vi "Facade.vi"(0 "Data In":T6, 2 "Display State In":T4, 3 "Container State":T5) -> (6 "Data Out":T6, 7 "Display State Out":T4, 8 "Action":T3)   [LabVIEW 2020, in "Channel.xctl"]
uses:
  Channel.xctl
  Data.vi
  Classes/Channel/Channel.lvclass
  <vilib>/_xctls/Container State.ctl
  State.vi
  <vilib>/_xctls/Action.ctl
  Waveforms/Waveform/Waveform.xctl
  Classes/Waveforms/Waveform/Waveform.lvclass
  D:/Development/epl-vi-lib/Koop/KObject Class/KObject.lvclass
  Level/Level.xctl
  Classes/Level/Level.lvclass
  Gate/Gate.xctl
  Classes/Gate/Gate.lvclass
  Filter/Filter.xctl
  Classes/Filter/Filter.lvclass
  Modulations/AM/AM.xctl
  Classes/Modulations/AM/AM.lvclass
  Utility VIs/Buttons/KCheckmarkBoolean 2.ctl
  Classes/Channel/Channel.lvclass/Channel.ctl
  Classes/Channel/Write Destination.vi
  Classes/Channel/Write Level.vi
  Classes/Channel/Write Filter.vi
  Classes/Channel/Write Gate.vi
  Classes/Channel/Write AM.vi
  Classes/Channel/Write Invert.vi
  Classes/Channel/Write AltPol.vi
  Classes/Channel/Write Persist.vi
  Classes/Channel/Read Waveform.vi
  Classes/Channel/Read Level.vi
  Classes/Channel/Read Gate.vi
  Classes/Channel/Read Filter.vi
  Classes/Channel/Read AM.vi
  Classes/Channel/Read Invert.vi
  Classes/Channel/Read AltPol.vi
  Classes/Channel/Read Persist.vi
  Classes/Channel/Read Destination.vi
  <vilib>/_xctls/XControlSupport.lvlib
  Koop/KObject Class/KObject.lvclass
panel:
  in  "Destination":u16(ring) caption="is"
  in  "Tabs":T1(tab)
  in  "Waveform":refnum<class "Waveform.lvclass">(xcontrol)
  in  "Filter":refnum<class "Filter.lvclass">(xcontrol)
  in  "Level":refnum<class "Level.lvclass">(xcontrol)
  in  "Gate":refnum<class "Gate.lvclass">(xcontrol)
  in  "AM":refnum<class "AM.lvclass">(xcontrol)
  in  "Fade out (ms)":dbl min=0.0
  in  "Fade in (ms)":dbl min=0.0
  in  "Persist":T2
  in  "Invert":T2
  in  "Alternate polarity":T2
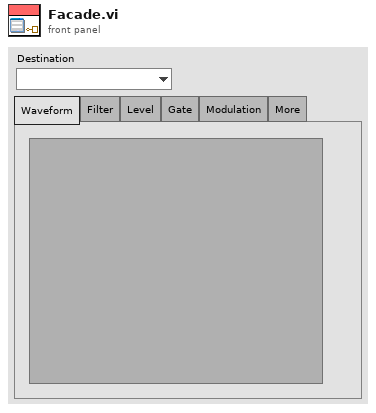
[diagram p1: front panel]
types:
  T1 = enum32{"Waveform", "Filter", "Level", "Gate", "Modulation", "More"}
  T2 = typedef "KCheckmarkBoolean 2.ctl" = bool
  T3 = typedef "XControlSupport.lvlib/Action.ctl" = cluster{"Data Changed?":bool, "State Changed?":bool, "Action Name":string}
  T4 = typedef "Channel.xctl/State.vi" = cluster{"action":string, "Destinations":string[]}
  T5 = typedef "XControlSupport.lvlib/Container State.ctl" = cluster{"Indicator?":bool, "Run Mode?":bool, " Refnum":refnum<vi>}
  T6 = typedef "Channel.xctl/Data.vi" = refnum<class "Channel.lvclass">
  T7 = typedef "Waveform.lvclass/Attributes.ctl" = cluster{"Spectrum":bool, "Gate":bool, "Mod":bool, "Filter":bool}
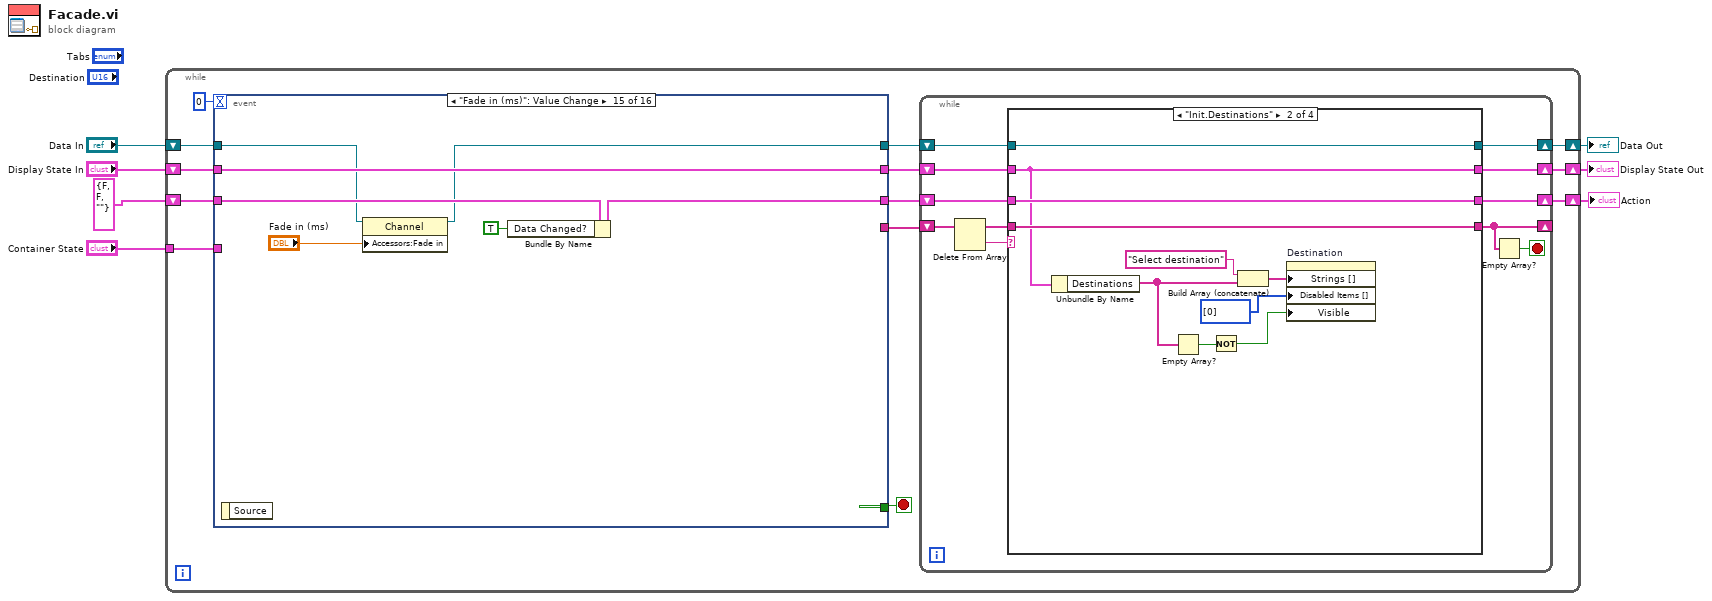
[diagram p0: block diagram]
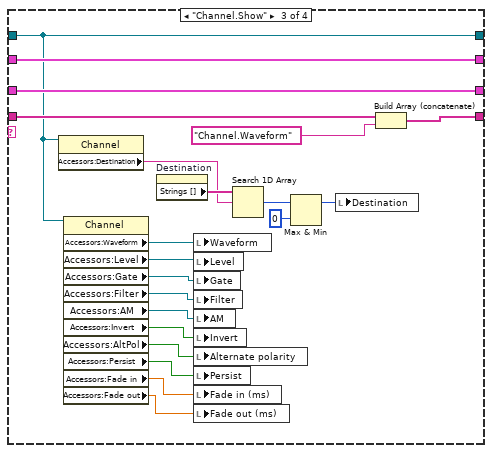
[diagram p3: hidden frame]
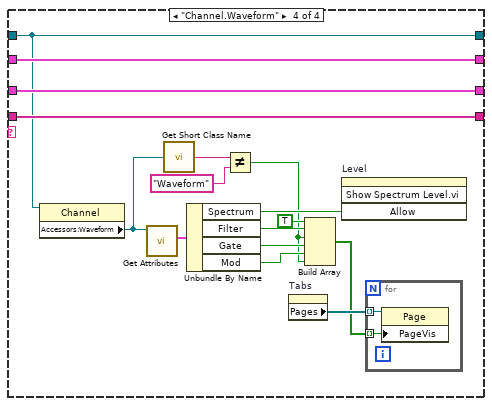
[diagram p4: hidden frame]
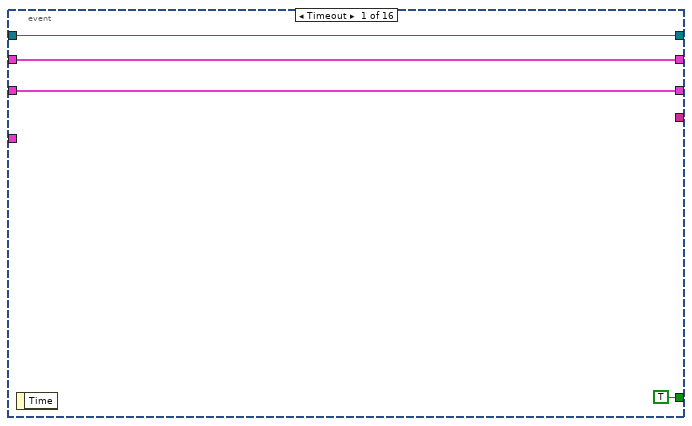
[diagram p5: hidden frame]
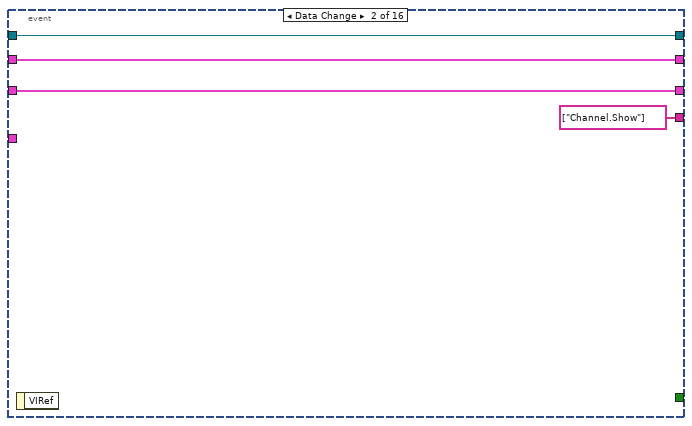
[diagram p6: hidden frame]
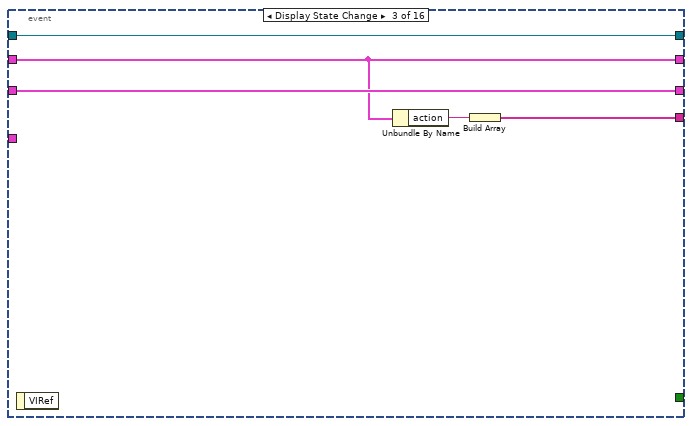
[diagram p7: hidden frame]
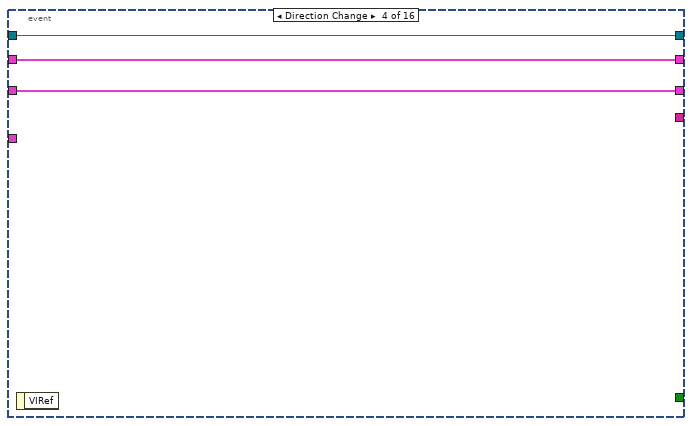
[diagram p8: hidden frame]
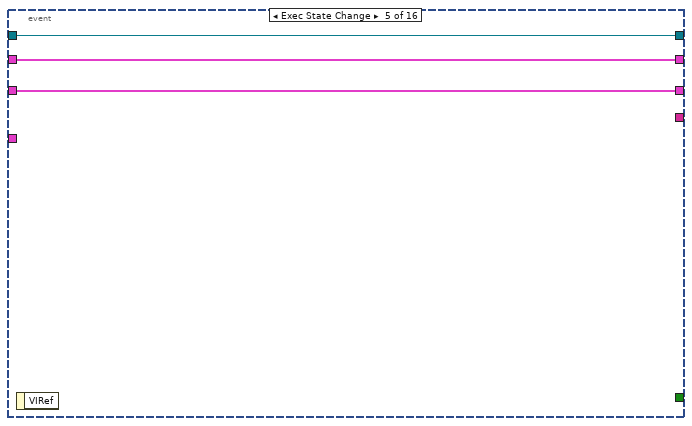
[diagram p9: hidden frame]
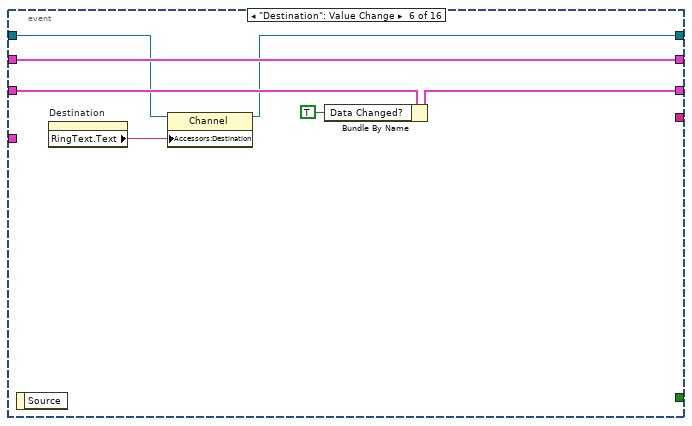
[diagram p10: hidden frame]
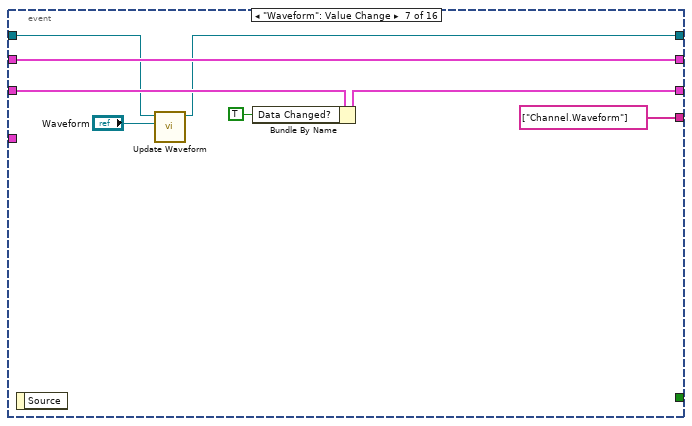
[diagram p11: hidden frame]
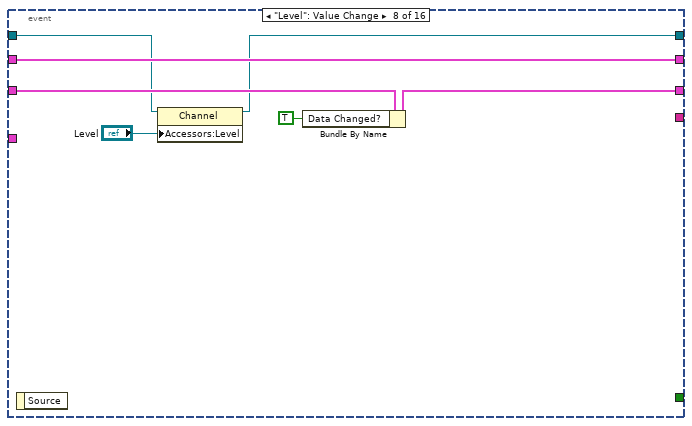
[diagram p12: hidden frame]
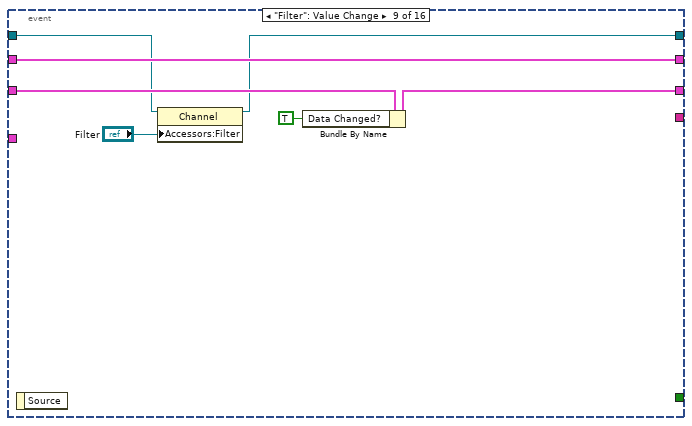
[diagram p13: hidden frame]
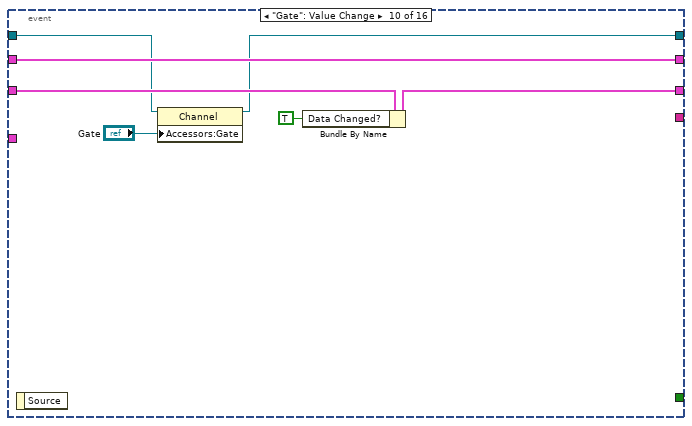
[diagram p14: hidden frame]
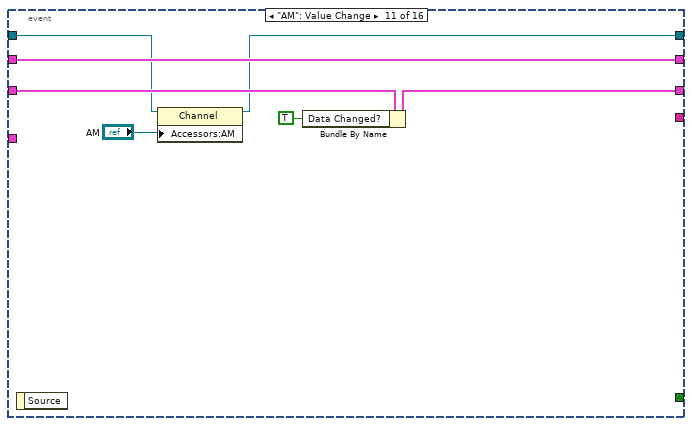
[diagram p15: hidden frame]
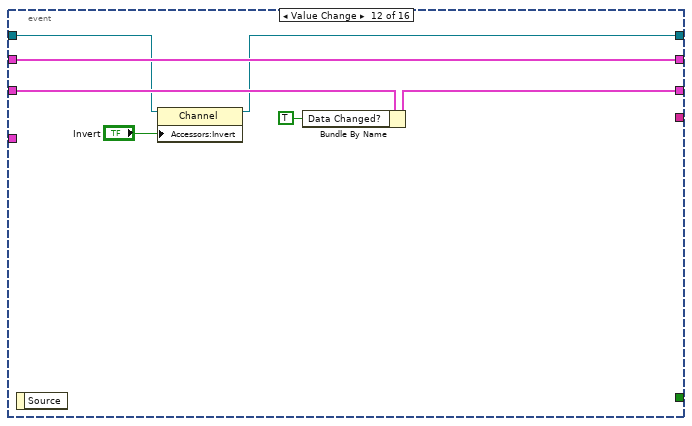
[diagram p16: hidden frame]
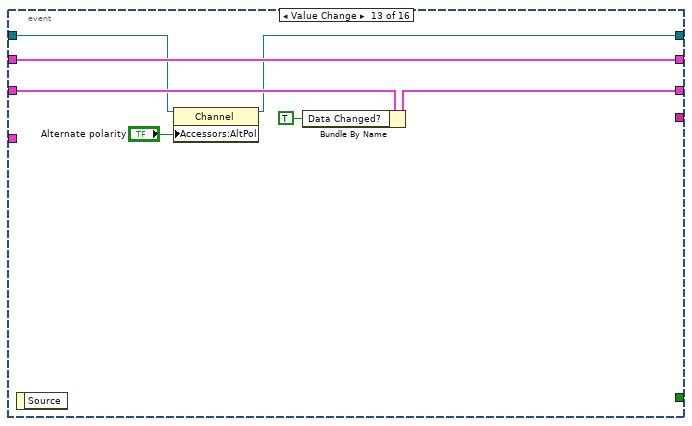
[diagram p17: hidden frame]
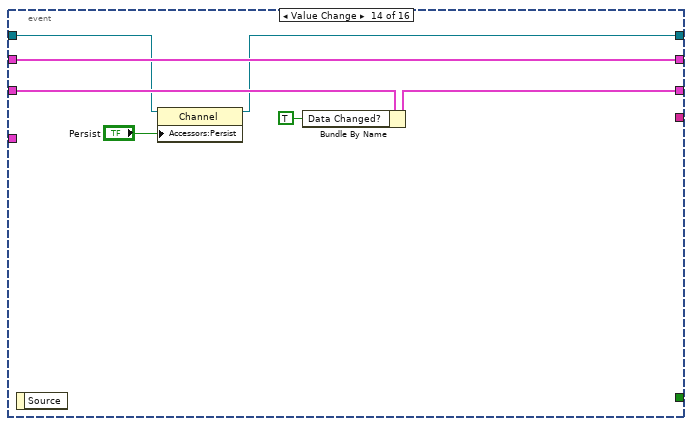
[diagram p18: hidden frame]
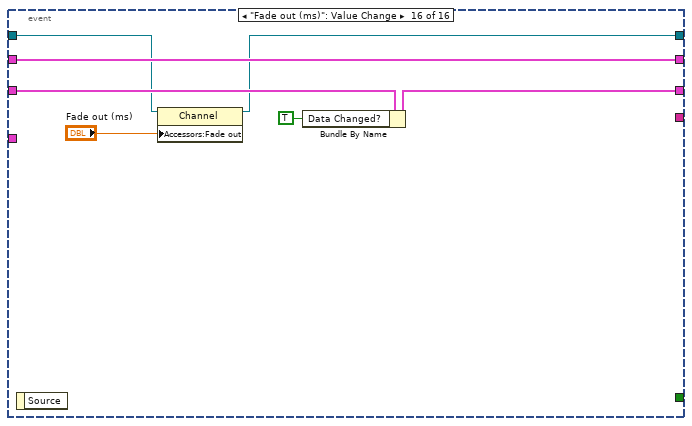
[diagram p19: hidden frame]
diagram:
  n1 = while {
    shift-right: [w9] -> w4
    shift-left: "Display State In" -> [w20]
    tunnel: "Container State" -> [w17]
    shift-right: [w10] -> w7
    shift-left: "Data In" -> [w16]
    shift-right: [w8] -> w2
    shift-left: T3 {"Data Changed?"=FALSE, "State Changed?"=FALSE, "Action Name"=""} ("Action") -> [w15]
    stop <- w19 stop-if-true
    n2 = event shown="[14] \"Fade in (ms)\": Value Change" {
      selector: _ -> [_ _ _ _ _ _ _ _ _ _ _ _ _ _ _ _]
      dyn-events: _ -> [_ _ _ _ _ _ _ _ _ _ _ _ _ _ _ _]
      timeout: 0 -> [_ _ _ _ _ _ _ _ _ _ _ _ _ _ _ _]
      tunnel: w20 -> [w86 w91 w95 w100 w103 w110 w118 w125 w132 w139 w146 w153 w160 w167 w174 w181]
      tunnel: [w86 w91 w95 w100 w103 w110 w118 w125 w132 w139 w146 w153 w160 w167 w174 w181] -> w12
      tunnel: [TRUE _ _ _ _ _ _ _ _ _ _ _ _ _ _ _] -> w19
      tunnel: w17 -> [_ _ _ _ _ _ _ _ _ _ _ _ _ _ _ _]
      tunnel: w16 -> [w85 w92 w97 w99 w102 w108 w114 w123 w130 w137 w144 w151 w158 w165 w172 w179]
      tunnel: [w85 w92 w97 w99 w102 w107 w113 w122 w129 w136 w143 w150 w157 w164 w171 w178] -> w13
      tunnel: [w87 w90 w96 w98 w101 w105 w116 w120 w128 w135 w142 w149 w156 w163 w170 w177] -> w11
      tunnel: w15 -> [w87 w90 w96 w98 w101 w109 w117 w124 w131 w138 w145 w152 w159 w166 w173 w180]
      tunnel: [_ string[] ["Channel.Show"] w93 _ _ _ string[] ["Channel.Waveform"] _ _ _ _ _ _ _ _ _] -> w14
      event Timeout {
        n3 = event-data() -> ()  [unwired: 1 in, 1 out]
      }
      event Data Change {
        n4 = event-data() -> ()  [unwired: 1 in, 1 out]
      }
      event Display State Change {
        n5 = event-data() -> ()  [unwired: 1 in, 1 out]
        n6 = Unbundle By Name(w95) -> ("action"=w94:string)
        n7 = Build Array(w94) -> (w93:string[])
      }
      event Direction Change {
        n8 = event-data() -> ()  [unwired: 1 in, 1 out]
      }
      event Exec State Change {
        n9 = event-data() -> ()  [unwired: 1 in, 1 out]
      }
      event "Destination": Value Change {
        n10 = event-data() -> ()  [unwired: 1 in, 1 out]
        n11 = property on="Destination" class="Ring (strict)"() -> ("RingText.Text"=w106:string)  [unwired: 2 in, 2 out]
        n12 = property class="Channel"(reference=w108, "Accessors:Destination"=w106) -> (reference out=w107:T6)  [unwired: 1 in, 1 out]
        n13 = Bundle By Name(cluster=w109, "Data Changed?"=TRUE) -> (w105:T3)
      }
      event "Waveform": Value Change {
        n14 = event-data() -> ()  [unwired: 1 in, 1 out]
        n15 = call "Update Waveform.vi"("Waveform"="Waveform", "Channel in"=w114) -> ("Channel out"=w113:T6)  [unwired: 8 in, 1 out]
        n16 = Bundle By Name(cluster=w117, "Data Changed?"=TRUE) -> (w116:T3)
      }
      event "Level": Value Change {
        n17 = event-data() -> ()  [unwired: 1 in, 1 out]
        n18 = property class="Channel"(reference=w123, "Accessors:Level"="Level") -> (reference out=w122:T6)  [unwired: 1 in, 1 out]
        n19 = Bundle By Name(cluster=w124, "Data Changed?"=TRUE) -> (w120:T3)
      }
      event "Filter": Value Change {
        n20 = event-data() -> ()  [unwired: 1 in, 1 out]
        n21 = property class="Channel"(reference=w130, "Accessors:Filter"="Filter") -> (reference out=w129:T6)  [unwired: 1 in, 1 out]
        n22 = Bundle By Name(cluster=w131, "Data Changed?"=TRUE) -> (w128:T3)
      }
      event "Gate": Value Change {
        n23 = event-data() -> ()  [unwired: 1 in, 1 out]
        n24 = property class="Channel"(reference=w137, "Accessors:Gate"="Gate") -> (reference out=w136:T6)  [unwired: 1 in, 1 out]
        n25 = Bundle By Name(cluster=w138, "Data Changed?"=TRUE) -> (w135:T3)
      }
      event "AM": Value Change {
        n26 = event-data() -> ()  [unwired: 1 in, 1 out]
        n27 = property class="Channel"(reference=w144, "Accessors:AM"="AM") -> (reference out=w143:T6)  [unwired: 1 in, 1 out]
        n28 = Bundle By Name(cluster=w145, "Data Changed?"=TRUE) -> (w142:T3)
      }
      event Value Change {
        n29 = event-data() -> ()  [unwired: 1 in, 1 out]
        n30 = property class="Channel"(reference=w151, "Accessors:Invert"="Invert") -> (reference out=w150:T6)  [unwired: 1 in, 1 out]
        n31 = Bundle By Name(cluster=w152, "Data Changed?"=TRUE) -> (w149:T3)
      }
      event Value Change {
        n32 = event-data() -> ()  [unwired: 1 in, 1 out]
        n33 = property class="Channel"(reference=w158, "Accessors:AltPol"="Alternate polarity") -> (reference out=w157:T6)  [unwired: 1 in, 1 out]
        n34 = Bundle By Name(cluster=w159, "Data Changed?"=TRUE) -> (w156:T3)
      }
      event Value Change {
        n35 = event-data() -> ()  [unwired: 1 in, 1 out]
        n36 = property class="Channel"(reference=w165, "Accessors:Persist"="Persist") -> (reference out=w164:T6)  [unwired: 1 in, 1 out]
        n37 = Bundle By Name(cluster=w166, "Data Changed?"=TRUE) -> (w163:T3)
      }
      event "Fade in (ms)": Value Change {
        n38 = event-data() -> ()  [unwired: 1 in, 1 out]
        n39 = property class="Channel"(reference=w172, "Accessors:Fade in"="Fade in (ms)") -> (reference out=w171:T6)  [unwired: 1 in, 1 out]
        n40 = Bundle By Name(cluster=w173, "Data Changed?"=TRUE) -> (w170:T3)
      }
      event "Fade out (ms)": Value Change {
        n41 = event-data() -> ()  [unwired: 1 in, 1 out]
        n42 = property class="Channel"(reference=w179, "Accessors:Fade out"="Fade out (ms)") -> (reference out=w178:T6)  [unwired: 1 in, 1 out]
        n43 = Bundle By Name(cluster=w180, "Data Changed?"=TRUE) -> (w177:T3)
      }
    }
    n44 = while {
      shift-right: [w28] -> _
      shift-left: w14 -> [w31]
      shift-right: [w26] -> w10
      shift-left: w13 -> [w25]
      shift-right: [w24] -> w9
      shift-left: w12 -> [w23]
      shift-right: [w22] -> w8
      shift-left: w11 -> [w21]
      stop <- w27 stop-if-true
      n45 = Delete From Array(array=w31) -> (deleted portion=w29:string, array with subset deleted=w30:string[])  [unwired: 2 in]
      n46 = case shown="\"Init.Destinations\"" w29 {
        tunnel: w30 -> [w35 w45 w66 w82]
        tunnel: [w35 w45 w56 w82] -> w28
        tunnel: [w34 w44 w58 w79] -> w26
        tunnel: w25 -> [w34 w44 w58 w79]
        tunnel: [w33 w42 w65 w81] -> w24
        tunnel: w23 -> [w33 w42 w65 w81]
        tunnel: [w32 w43 w64 w80] -> w22
        tunnel: w21 -> [w32 w43 w64 w80]
        frame "", Default {
        }
        frame "Init.Destinations" {
          n47 = Unbundle By Name(w42) -> ("Destinations"=w38:string[])
          n48 = Empty Array?(array=w38) -> (empty?=w37:bool)
          n49 = Not(x=w37) -> (.not. x?=w36:bool)
          n50 = Build Array (concatenate)("Select destination", w38) -> (w41:string[])
          n51 = property on="Destination" class="Ring (strict)"("Strings []"=w41, "Disabled Items []"=i32[] [0], "Visible"=w36) -> ()  [unwired: 2 in, 2 out]
        }
        frame "Channel.Show" {
          n52 = property class="Channel"(reference=w58) -> ("Accessors:Destination"=w62:string)  [unwired: 1 in, 2 out]
          n53 = property class="Channel"(reference=w58) -> ("Accessors:Waveform"=w57:refnum<class "Waveform.lvclass">, "Accessors:Level"=w54:refnum<class "Level.lvclass">, "Accessors:Gate"=w53:refnum<class "Gate.lvclass">, "Accessors:Filter"=w52:refnum<class "Filter.lvclass">, "Accessors:AM"=w51:refnum<class "AM.lvclass">, "Accessors:Invert"=w50:bool, "Accessors:AltPol"=w49:bool, "Accessors:Persist"=w48:bool, "Accessors:Fade in"=w47:dbl, "Accessors:Fade out"=w46:dbl)  [unwired: 1 in, 2 out]
          n54 = property on="Destination" class="Ring (strict)"() -> ("Strings []"=w63:string[])  [unwired: 2 in, 2 out]
          n55 = local write "Waveform"(w57) -> ()
          n56 = local write "Level"(w54) -> ()
          n57 = local write "Gate"(w53) -> ()
          n58 = local write "Filter"(w52) -> ()
          n59 = local write "AM"(w51) -> ()
          n60 = local write "Invert"(w50) -> ()
          n61 = local write "Alternate polarity"(w49) -> ()
          n62 = local write "Persist"(w48) -> ()
          n63 = local write "Fade in (ms)"(w47) -> ()
          n64 = local write "Fade out (ms)"(w46) -> ()
          n65 = Search 1D Array(1D array=w63, element=w62) -> (index of element=w61:i32)  [unwired: 1 in]
          n66 = Max & Min(x=w61, y=0) -> (max(x,y)=w59:i32)  [unwired: 1 out]
          n67 = local write "Destination"(w59) -> ()
          n68 = Build Array (concatenate)(w66, "Channel.Waveform") -> (w56:string[])
        }
        frame "Channel.Waveform" {
          n69 = property class="Channel"(reference=w79) -> ("Accessors:Waveform"=w70:refnum<class "Waveform.lvclass">)  [unwired: 1 in, 2 out]
          n70 = call-dynamic "Get Attributes.vi"("Waveform in"=w70) -> ("Attributes"=w78:T7)  [unwired: 8 in, 2 out]
          n71 = call "Get Short Class Name.vi"("KObject in"=w70) -> ("Class"=w69:string)  [unwired: 4 in]
          n72 = Unbundle By Name(w78) -> ("Spectrum"=w77:bool, "Filter"=w76:bool, "Gate"=w75:bool, "Mod"=w74:bool)
          n73 = Not Equal?(x=w69, y="Waveform") -> (x != y?=w67:bool)
          n74 = property on="Tabs" class="TabCtl (strict)"() -> ("Pages"=w72:refnum<vi>[])  [unwired: 2 in, 2 out]
          n75 = Build Array(TRUE, w76, w67, w75, w74, w67) -> (w71:bool[])
          n76 = invoke on="Level" class="Level (strict)" method="Show Spectrum Level.vi"("Allow"=w77) -> ()  [unwired: 3 in, 4 out]
          n77 = for {
            tunnel: w72 -> [w84] mode=indexing
            tunnel: w71 -> [w83] mode=indexing
            n78 = property class="Page"(reference=w84, "PageVis"=w83) -> ()  [unwired: 1 in, 2 out]
          }
        }
      }
      n79 = Empty Array?(array=w28) -> (empty?=w27:bool)
    }
  }
  "Display State Out" <- w4
  "Data Out" <- w7
  "Action" <- w2
